vi "AVS_go_Remote.vi"(2 "RANGE  (-1:no change)":i8=-1 min=-1 max=7) -> (0 "error out":errorcluster, 1 "dup VISA session":refnum<visa-resource-name>)   [LabVIEW 2010]
uses:
  ControlCentre/Global 1.vi
  Programme/National Instruments/LabVIEW 8.5/instr.lib/Mischerinstr.lib/AVS-Brücke/LV Drivers for AVS/AVS47IB.LLB/AVS47IB Wait for OPC/MAV/TMO.vi
panel:
  in  "error in (no error)":errorcluster
  in  "Delay (sec)":i16=1 min=0 max=3600 step=1
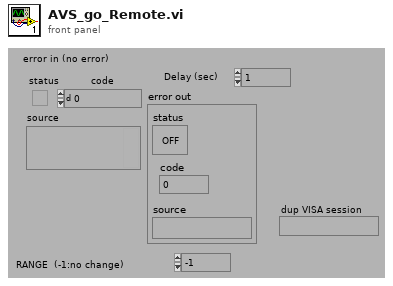
[diagram p1: front panel]
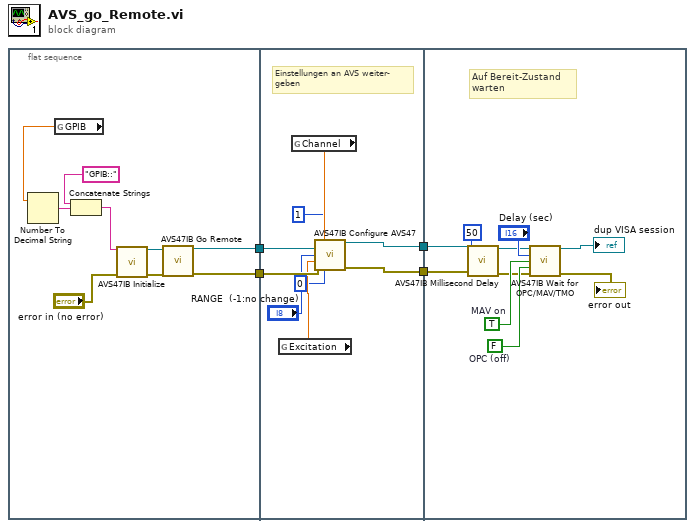
[diagram p0: block diagram]
diagram:
  n1 = flat-sequence {
    tunnel: [w6] -> w4
    tunnel: [w5] -> w3
    tunnel: w4 -> [w22]
    tunnel: w3 -> [w21]
    tunnel: [w20] -> w2
    tunnel: [w19] -> w1
    tunnel: w2 -> [w26]
    tunnel: w1 -> [w25]
    frame #0 {
      n2 = global read "Global 1.vi" "GPIB"() -> (w9:dbl)
      n3 = Number To Decimal String(number=w9) -> (decimal integer string=w12:string)  [unwired: 1 in]
      n4 = Concatenate Strings("GPIB::", w12) -> (w10:string)
      n5 = call "AVS47IB Initialize.vi"("Instr. Descriptor (GPIB::)"=w10, "error in (no error)"="error in (no error)") -> ("VISA session"=w8:refnum<visa-resource-name>, "error out"=w7:errorcluster)  [unwired: 12 in]
      n6 = call "AVS47IB Go Remote.vi"("VISA session"=w8, "error in (no error)"=w7) -> ("dup VISA session"=w6:refnum<visa-resource-name>, "error out"=w5:errorcluster)  [unwired: 12 in]
    }
    frame #1 {
      # "Einstellungen an AVS weiter-\ngeben"
      n7 = global read "Global 1.vi" "Excitation"() -> (w17:dbl)
      n8 = global read "Global 1.vi" "Channel"() -> (w18:dbl)
      n9 = call "AVS47IB Configure AVS47.vi"("VISA session"=w22, "INPUT (-1:no change)"=i8 1, "CHANNEL (-1:no change )"=w18, "RANGE  (-1:no change)"="RANGE  (-1:no change)", "EXCITATION (-1:no change)"=w17, "error in (no error)"=w21, "DISPLAY (-1:no change)"=i8 0) -> ("dup VISA session"=w20:refnum<visa-resource-name>, "error out"=w19:errorcluster)  [unwired: 7 in]
    }
    frame #2 {
      w31 = FALSE  # OPC (off)
      w32 = TRUE  # MAV on
      # "Auf Bereit-Zustand\nwarten"
      n10 = call "AVS47IB Millisecond Delay.vi"("VISA session"=w26, "Delay (50 ms)"=50, "error in (no error)"=w25) -> ("dup VISA session"=w29:refnum<visa-resource-name>, "error out"=w28:errorcluster)  [unwired: 11 in]
      n11 = call "AVS47IB Wait for OPC/MAV/TMO.vi"("VISA session"=w29, "Timeout (2 sec)"="Delay (sec)", "MAV (on)"=w32, "OPC (off)"=w31, "error in (no error)"=w28) -> ("dup VISA session"=→"dup VISA session":refnum<visa-resource-name>, "error out"=→"error out":errorcluster)  [unwired: 8 in, 1 out]
    }
  }
